vi "Connect_to_BSA_F600.vi"(3 "BSA IP Number":string="10.10.100.130") -> (0 "error out":errorcluster, 1 "F600":refnum<k7>)   [LabVIEW 2020]
uses:
  Globals/LDA_global.vi
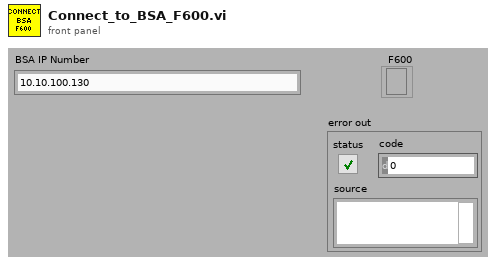
[diagram p1: front panel]
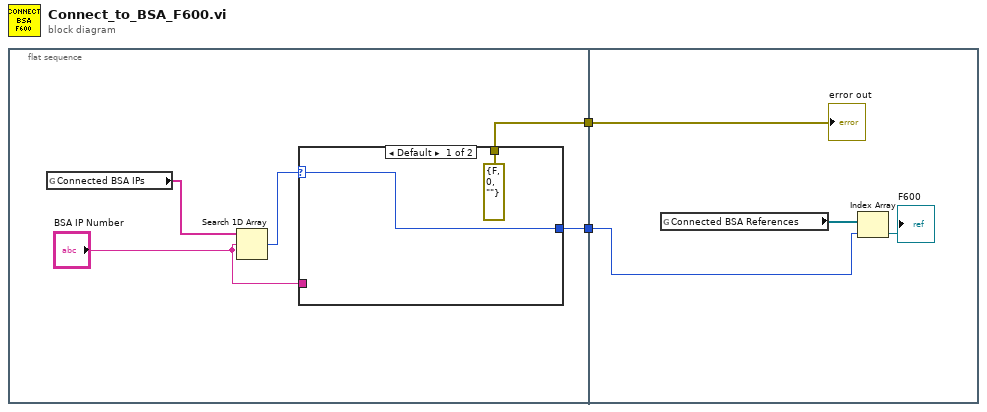
[diagram p0: block diagram]
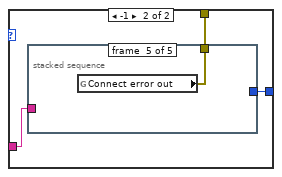
[diagram p2: hidden frame]
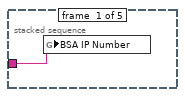
[diagram p3: hidden frame]
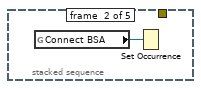
[diagram p4: hidden frame]
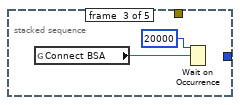
[diagram p5: hidden frame]
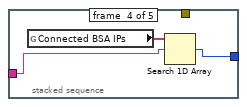
[diagram p6: hidden frame]
diagram:
  n1 = flat-sequence {
    tunnel: [w4] -> w2
    tunnel: [w3] -> w1
    tunnel: w2 -> [w22]
    tunnel: w1 -> [w21]
    frame #0 {
      n2 = global read "LDA_global.vi" "Connected BSA IPs"() -> (w5:string[])
      n3 = Search 1D Array(1D array=w5, element="BSA IP Number") -> (index of element=w6:i32)  [unwired: 1 in]
      n4 = case shown="Default" w6 {
        selector: w6 -> [w9 _]
        tunnel: "BSA IP Number" -> [_ w12]
        tunnel: [w9 w11] -> w4
        tunnel: [errorcluster {"status"=FALSE, "code"=0, "source"=""} ("Connect error out") w10] -> w3
        frame Default {
        }
        frame -1 {
          n5 = stacked-sequence {
            tunnel: w12 -> [w13 _ _ w17 _]
            tunnel: [_ _ _ w18 _] -> w11
            tunnel: [_ _ _ _ w20] -> w10
            frame #0 {
              n6 = global write "LDA_global.vi" "BSA IP Number"(w13) -> ()
            }
            frame #1 {
              n7 = global read "LDA_global.vi" "Connect BSA"() -> (w14:refnum<k4>)
              n8 = Set Occurrence(w14) -> ()
            }
            frame #2 {
              n9 = global read "LDA_global.vi" "Connect BSA"() -> (w16:refnum<k4>)
              n10 = Wait on Occurrence(2:w16, 3:20000 ("ms timeout (-1)")) -> ()  [unwired: 2 out]
            }
            frame #3 {
              n11 = global read "LDA_global.vi" "Connected BSA IPs"() -> (w19:string[])
              n12 = Search 1D Array(1D array=w19, element=w17) -> (index of element=w18:i32)  [unwired: 1 in]
            }
            frame #4 {
              n13 = global read "LDA_global.vi" "Connect error out"() -> (w20:errorcluster)
            }
          }
        }
      }
    }
    frame #1 {
      n14 = global read "LDA_global.vi" "Connected BSA References"() -> (w24:refnum<k7>[])
      n15 = Index Array(array=w24, index=w22) -> (element=→"F600":refnum<k7>)
      "error out" <- w21
    }
  }
